vi "Populate Device Settings.vi"(8 "error in":errorcluster, 11 "UI Actor in":refnum<class "UI Actor.lvclass">) -> (0 "error out":errorcluster, 3 "UI Actor out":refnum<class "UI Actor.lvclass">)   [LabVIEW 2024, in "UI Actor.lvlib" / "UI Actor.lvclass"]
uses:
  UI Actor.lvclass
  Controls/Device Settings.ctl
  UI Actor.lvclass/UI Actor.ctl
  Core/Device Info/Device Info.lvclass
  Core/EDS/EDS.lvclass
  <vilib>/Utility/Data Type/NI_Data Type.lvlib
  <userlib>/_OpenG.lib/lvdata/lvdata.llb/openg_variant.lvlib
  <vilib>/JDP Science/JDP Science Common Utilities/JDP Utility.lvlib
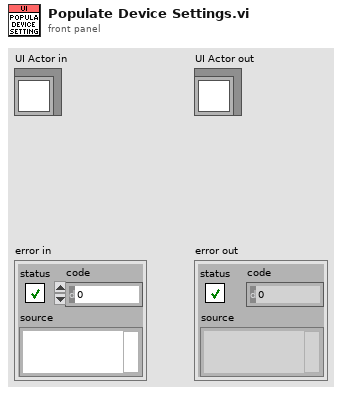
[diagram p1: front panel]
types:
  T1 = typedef "Device Settings.ctl" = cluster{"SimpleBootUpSlave":bool, "SimpleBootUpMaster":bool}
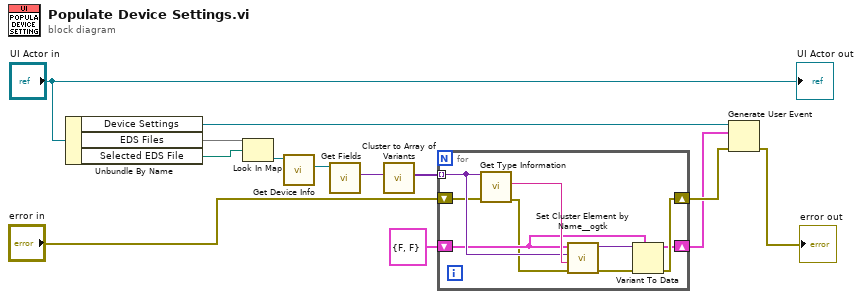
[diagram p0: block diagram]
diagram:
  n1 = Unbundle By Name("UI Actor in") -> ("Device Settings"=w12:refnum<user-event>, "EDS Files"=w10:map{path, refnum<class "EDS.lvclass">}, "Selected EDS File"=w9:path)
  n2 = Look In Map(map=w10, key=w9) -> (value=w6:refnum<class "EDS.lvclass">)  [unwired: 1 in, 1 out]
  n3 = call "Get Device Info.vi"("EDS in"=w6) -> ("Device Info"=w5:refnum<class "Device Info.lvclass">)  [unwired: 9 in, 1 out]
  n4 = call-dynamic "Get Fields.vi"("Device Info in"=w5) -> ("Fields Cluster"=w8:variant)  [unwired: 9 in, 1 out]
  n5 = call <vilib>:"Cluster to Array of Variants.vi"("Cluster"=w8) -> ("Array of Cluster Elements"=w7:variant[])  [unwired: 10 in]
  n6 = for {
    tunnel: w7 -> [w21] mode=indexing
    shift-right: [w16] -> w2
    shift-left: T1 {"SimpleBootUpSlave"=FALSE, "SimpleBootUpMaster"=FALSE} ("Device Settings") -> [w17]
    shift-right: [w19] -> w3
    shift-left: "error in" -> [w15]
    n7 = call <vilib>:"Get Type Information.vi"("error in (no error)"=w15, "variant"=w21) -> ("error out"=w14:errorcluster, "name"=w22:string)  [unwired: 5 in, 3 out]
    n8 = call <userlib>:"Set Cluster Element by Name__ogtk.vi"("error in (no error)"=w14, "Element Name (\"\": New Element Data Name)"=w22, "New Element Value"=w21, "Cluster"=w17) -> ("error out"=w20:errorcluster, "VCluster out"=w18:variant)  [unwired: 5 in, 1 out]
    n9 = Variant To Data(error in=w20, type=w17, Variant=w18) -> (data=w16:T1, error out=w19:errorcluster)
  }
  n10 = Generate User Event(user event=w12, event data cluster=w2, error in=w3) -> (error out=→"error out":errorcluster)  [unwired: 1 in, 1 out]
  "UI Actor out" <- "UI Actor in"
